vi "2DBoolRandomArray.vi"(10 "j":i32, 11 "i":i32) -> (2 "Main Board":T1[][](array[typedef]))   [LabVIEW 2020]
doc: "Create \"random\" 2D boolean array."
uses:
  Ctrls/ElementalCell.ctl
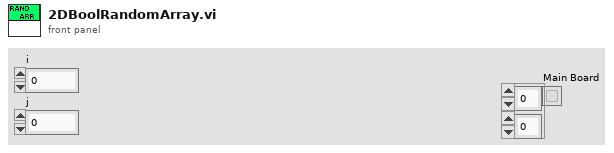
[diagram p1: front panel]
types:
  T1 = typedef "ElementalCell.ctl" = bool
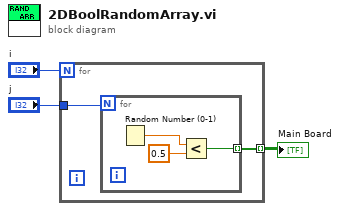
[diagram p0: block diagram]
diagram:
  n1 = for {
    N: "i" -> [_]
    tunnel: [w5] -> w3 mode=indexing
    tunnel: "j" -> [w4]
    n2 = for {
      N: w4 -> [_]
      tunnel: [w6] -> w5 mode=indexing
      n3 = Random Number (0-1)() -> (number: 0 to 1=w8:dbl)
      n4 = Less?(x=w8, y=0.5) -> (x < y?=w6:bool)
    }
  }
  "Main Board" <- w3
